vi "GetStatusParkerX.vi"(0 "Channel Properties":T1={"Channel Name"="", "Vel. Default"=5.0, "Acc. Default"=5.0, "Vel. Max"=5.0, "Vel. Min"=5.0, "Acc. Max"=5.0, "Acc. Min"=5.0, "Pulses/unit"=0.0, "Address"=0, "Pulse Offset"=0, "Pos Tolerance"=0.0, "Pulses/rev"=0.0, "Backlash/Eng units"=0.0, "Current Pos"=0.0, "Ch Status"=enum."Active", "Port Name"="", "Axis Transform mode"="", "Metadata Ch Name"="", "Type"=""} {"Current Pos" format="%.2f"; "Backlash/Eng units" format="%.2f"; "Pulses/rev" format="%.2f"; "Pos Tolerance" format="%.2f"; "Pulses/unit" format="%.2f"; "Acc. Min" format="%.2f"; "Acc. Max" format="%.2f"; "Vel. Min" format="%.2f"; "Vel. Max" format="%.2f"; "Acc. Default" format="%.2f"; "Vel. Default" format="%.2f"}, 2 "Limit switch valid?":bool, 3 "Stop on Trigger 3?":bool) -> (5 "Ready":bool, 6 "OK":bool, 7 "Position in Move":dbl format="%.2f", 8 "Error string":string)   [LabVIEW 2012]
uses:
  ~subVIs/DriveProperties.ctl
  X-_commands.ctl
panel:
  out "Output 2":i32
  out "Output 1":i32 format="%.0b"
  out "Remaining String":string
  out "CCW limit":bool
  out "Home":bool
  out "NOT FAULT":bool
  out "CCW limit":bool
  out "CW limit":bool
  out "Seq3":bool
  out "Seq2":bool
  out "Seq1":bool
  out "Trg3":bool
  out "Trg2":bool
  out "Trg1":bool
  out "Good Home":bool
  out "Stall":bool
  out "Trigger":bool
  out "Shutdown":bool
  out "Pausing":bool
  out "Looping":bool
  out "CW limit":bool
  out "Status":string
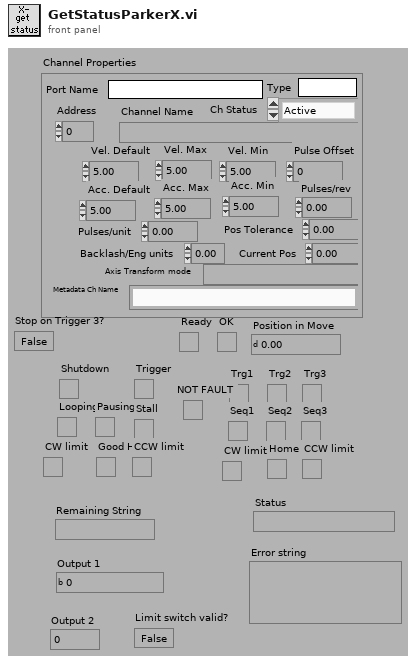
[diagram p1: front panel]
types:
  T1 = typedef "DriveProperties.ctl" = cluster{"Channel Name":string, "Vel. Default":dbl, "Acc. Default":dbl, "Vel. Max":dbl, "Vel. Min":dbl, "Acc. Max":dbl, "Acc. Min":dbl, "Pulses/unit":dbl, "Address":u8, "Pulse Offset":i32, "Pos Tolerance":dbl, "Pulses/rev":dbl, "Backlash/Eng units":dbl, "Current Pos":dbl, "Ch Status":enum16{"Active", "Offline", "Simulate"}, "Port Name":string, "Axis Transform mode":string, "Metadata Ch Name":string, "Type":string}
  T2 = typedef "X-_commands.ctl" = enum16{"A-    Acceleration (rps)", "B-    Buffer Status", "C-    Continue", "CG-  Correction Gain", "CR-  Cariage Return", "D-    Distance (pulses)", "DB-  Dead Band (encoder steps)", "DW- Deadband Window (encoder steps)", "E-    Enable Communications", "ER-  Encoder Resolution (steps/rev)", "F-    Disable Communications", "FS-  Encoder Functions Report", "FSA- Incremental/Absolute (0/1)", "FSB- Motor/Encoder Step Mode (0/1)", "FSC- Enable/Disable Position Maint. (1/0)", "FSD- Stop/Continue on Stall (1/0)", "FSE- Activate o/p1 on Stall (1/0)", "FSF- Stop Motion on Trig3 (1/0)", "FSG- Activate o/p2 in Deadband (1/0)", "FSH- Enable Stall Detect (1/0)", "G- Go", "GH- Go Home and Zero (+/-V)", "^H- Delete ", "H- Direction Reverse/CCW/CW (0,1,2)", "IS- Input Status", "K- Kill", "L- Loop (n)", "LD- Limit DISABLE (0-none,1-CW,2-CCW,3-Both)", "LF- Line Feed", "MC- Mode Continuous", "MN- Mode Normal", "MPA- Motor Postion Absolute", "MPI- Motor Position Incremental", "MR- Motor Resolution (Drive Steps/rev)", "N- End of Loop", "O- Output (00,01,10,11)", "OS- Report Homing Setup", "OSA- NO/NC Limits (1/0)", "OSB- Back Up to Home/Edge? (0/1)", "OSC- NO/NC Home Switch (1/0)", "OSD- Enable Encoder Z for Home (0/1)", "OSH- Reference Edge for Home CW/CCW (0/1)", "PR- Report ABSOLUTE Position", "PS- Pause until Continue", "PX- Report Absolute ENCODER Position", "PZ- Zero Absolute Counter", "\"- Quote (17 ASCII +Space)", "Q- Enter/Exit Velocity Profiling (1/0)", "R- Request Indexer Status", "RA- Report Limit Switch Status", "RB- Report Loop, Pause, Shutdown, Trigger Status", "RC- Report Closed Loop Status", "RM- Velocity Streaming Rate Multiplier (000-FFF)", "RV- Report Revision Level", "S- Controlled Stop", "SN- Debounce (1-1000ms)", "SS- Report Software Switch Status", "SSA- Disable RS232 Echo (1/0)", "SSG- Clear/Save Command Buffer on Limit (0/1)", "SSH- Clear/Save Command Buffer on Stop (0/1)", "ST- Shutdown (1/0)", "SV- Servoing Setting (0,1,2,3)", "T- Time Delay (0.01-99999.99)", "TR- Wait for Trigger High/Low/Ignore (1/0/X)", "TS- Report Trigger Status", "U- Pause after Move Until Continue", "V- Velocity (0.01-50.00 revs/sec)", "W1- Report Relative Position <Signed Binary>", "W3- Report Relative Position <Hexadecimal>", "Y- Abort Loop at N", "Z-    Reset to Defaults", "#-    Disable/Set Soft Addresses (0/1-255)"}
  T3 = cluster{"Boolean array[0]":bool, "Boolean array[1]":bool, "Boolean array[2]":bool, "Boolean array[3]":bool}
  T4 = cluster{"Boolean array[0]":bool, "Boolean array[1]":bool, "Boolean array[2]":bool, "Boolean array[3]":bool, "Boolean array[4]":bool, "Boolean array[5]":bool, "Boolean array[6]":bool, "Boolean array[7]":bool, "Boolean array[8]":bool, "Boolean array[9]":bool}
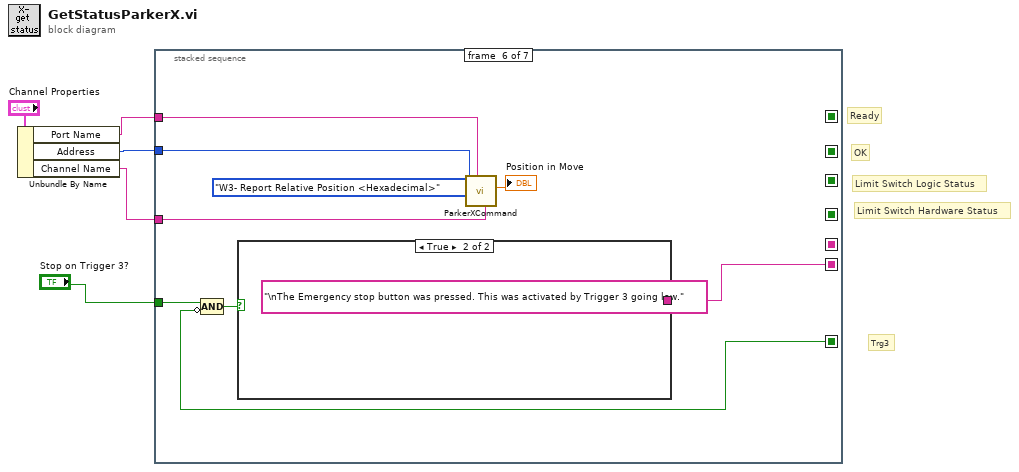
[diagram p0: block diagram]
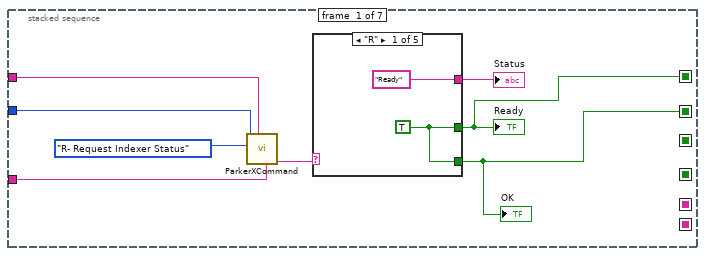
[diagram p2: hidden frame]
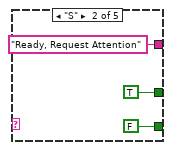
[diagram p3: hidden frame]
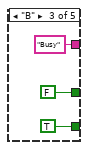
[diagram p4: hidden frame]
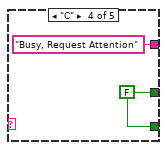
[diagram p5: hidden frame]
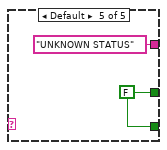
[diagram p6: hidden frame]
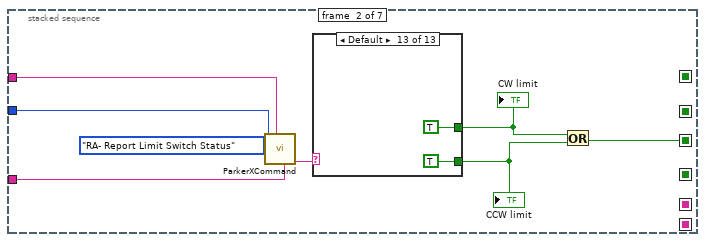
[diagram p7: hidden frame]
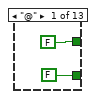
[diagram p8: hidden frame]
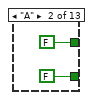
[diagram p9: hidden frame]
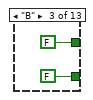
[diagram p10: hidden frame]
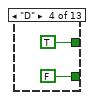
[diagram p11: hidden frame]
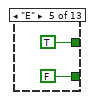
[diagram p12: hidden frame]
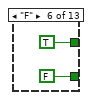
[diagram p13: hidden frame]
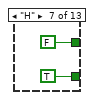
[diagram p14: hidden frame]
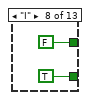
[diagram p15: hidden frame]
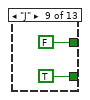
[diagram p16: hidden frame]
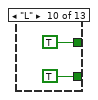
[diagram p17: hidden frame]
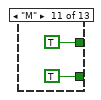
[diagram p18: hidden frame]
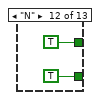
[diagram p19: hidden frame]
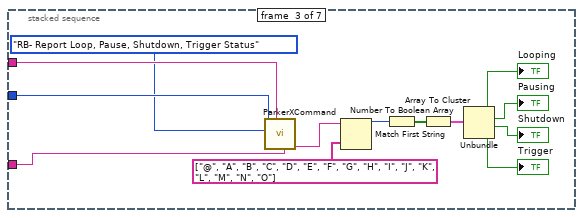
[diagram p20: hidden frame]
diagram:
  # "Trg3"
  # "Limit Switch Hardware Status"
  # "Limit Switch Logic Status"
  # "Ready"
  # "OK"
  n1 = Unbundle By Name("Channel Properties") -> ("Port Name"=w5:string, "Address"=w4:u8, "Channel Name"=w3:string)
  n2 = stacked-sequence {
    seq-local: [_ _ _ _ w94 _ _] -> [_ _ _ _ _ _ w138]
    seq-local: [_ w26 _ _ _ _ _] -> [_ _ _ _ _ _ w139]
    seq-local: [w8 _ _ _ _ _ _] -> [_ _ _ _ _ _ _]
    seq-local: [_ _ _ w73 _ _ _] -> [_ _ _ _ _ _ w146]
    seq-local: [w6 _ _ _ _ _ _] -> [_ _ _ _ _ _ w140]
    seq-local: [_ _ _ _ w93 _ _] -> [_ _ _ _ _ w126 _]
    seq-local: [_ _ _ _ _ w128 _] -> [_ _ _ _ _ _ w136]
    tunnel: w4 -> [w13 w33 w72 w82 w97 w133 _]
    tunnel: w5 -> [w7 w32 w71 w81 w96 w132 _]
    tunnel: w3 -> [w9 w29 w60 w77 w95 w129 w141]
    tunnel: "Stop on Trigger 3?" -> [_ _ _ _ w92 w127 _]
    frame #0 {
      n3 = call "ParkerXCommand.vi"("Channel Name"=w9, "Port Name"=w7, "COMMAND"=X-_commands."R- Request Indexer Status", "Address"=w13) -> ("String Reply"=w12:string)  [unwired: 3 in, 3 out]
      n4 = case shown="\"R\"" w12 {
        tunnel: ["Ready" "Ready, Request Attention" "Busy" "Busy, Request Attention" "UNKNOWN STATUS"] -> w11
        tunnel: [w14 TRUE FALSE w22 w24] -> w6
        tunnel: [w14 FALSE TRUE w22 w24] -> w8
        frame "R" {
          w14 = TRUE
        }
        frame "S" {
        }
        frame "B" {
        }
        frame "C" {
          w22 = FALSE
        }
        frame Default {
          w24 = FALSE
        }
      }
      "Status" <- w11
      "Ready" <- w6
      "OK" <- w8
    }
    frame #1 {
      n5 = call "ParkerXCommand.vi"("Channel Name"=w29, "Port Name"=w32, "COMMAND"=X-_commands."RA- Report Limit Switch Status", "Address"=w33) -> ("String Reply"=w31:string)  [unwired: 3 in, 3 out]
      n6 = case shown="Default" w31 {
        tunnel: [FALSE FALSE FALSE TRUE TRUE TRUE FALSE FALSE FALSE TRUE TRUE TRUE TRUE] -> w28
        tunnel: [FALSE FALSE FALSE FALSE FALSE FALSE TRUE TRUE TRUE TRUE TRUE TRUE TRUE] -> w27
        frame "@" {
        }
        frame "A" {
        }
        frame "B" {
        }
        frame "D" {
        }
        frame "E" {
        }
        frame "F" {
        }
        frame "H" {
        }
        frame "I" {
        }
        frame "J" {
        }
        frame "L" {
        }
        frame "M" {
        }
        frame "N" {
        }
        frame Default {
        }
      }
      "CW limit" <- w28
      "CCW limit" <- w27
      n7 = Or(x=w28, y=w27) -> (x .or. y?=w26:bool)
    }
    frame #2 {
      n8 = call "ParkerXCommand.vi"("Channel Name"=w60, "Port Name"=w71, "COMMAND"=X-_commands."RB- Report Loop, Pause, Shutdown, Trigger Status", "Address"=w72) -> ("String Reply"=w69:string)  [unwired: 3 in, 3 out]
      n9 = Match First String(2:string[] ["@", "A", "B", "C", "D", "E", "F", "G", "H", "I", "J", "K", "L", "M", "N", "O"], 3:w69) -> (0:w67:i32)  [unwired: 1 out]
      n10 = Number To Boolean Array(number=w67) -> (Boolean array=w66:bool[])
      n11 = Array To Cluster(array=w66) -> (cluster=w65:T3)
      n12 = Unbundle(w65) -> ("Boolean array[0]"=→"Looping":bool, "Boolean array[1]"=→"Pausing":bool, "Boolean array[2]"=→"Shutdown":bool, "Boolean array[3]"=→"Trigger":bool)
    }
    frame #3 {
      n13 = call "ParkerXCommand.vi"("Channel Name"=w77, "Port Name"=w81, "COMMAND"=X-_commands."RC- Report Closed Loop Status", "Address"=w82) -> ("String Reply"=w79:string)  [unwired: 3 in, 3 out]
      n14 = case shown="\"B\"" w79 {
        tunnel: [FALSE TRUE FALSE TRUE w91] -> w74
        tunnel: [TRUE TRUE FALSE FALSE w91] -> w78
        frame "@" {
        }
        frame "A" {
        }
        frame "B" {
        }
        frame "C" {
        }
        frame Default {
          w91 = FALSE
          (unwired) "UNKNOWN STATUS"
        }
      }
      "Stall" <- w74
      "Good Home" <- w78
      n15 = Select(t=" Motor Stalled", s=w74, f="") -> (s? t:f=w73:string)
    }
    frame #4 {
      n16 = while {
        tunnel: w97 -> [w124]
        tunnel: w96 -> [w123]
        tunnel: w95 -> [w121]
        tunnel: [w104] -> w94
        tunnel: [w103] -> w93
        tunnel: w92 -> [w98]
        i -> [w102]
        stop <- w99 continue-if-true
        n17 = call "ParkerXCommand.vi"("Channel Name"=w121, "Port Name"=w123, "COMMAND"=X-_commands."IS- Input Status", "Address"=w124) -> ("String Reply"=w120:string)  [unwired: 3 in, 3 out]
        n18 = Scan From String(format string="%10b%1d" ("Format String"), input string=w120) -> (remaining string=→"Remaining String":string, output 1=w116:i32, output 2=→"Output 2":i32)  [unwired: 2 in, 4 out]
        "Output 1" <- w116
        n19 = Less?(x=w102, y=3) -> (x < y?=w100:bool)
        n20 = Number To Boolean Array(number=w116) -> (Boolean array=w115:bool[])
        n21 = Array To Cluster(array=w115) -> (cluster=w114:T4)
        n22 = Unbundle(w114) -> ("Boolean array[0]"=→"Seq3":bool, "Boolean array[1]"=→"Seq2":bool, "Boolean array[2]"=→"Seq1":bool, "Boolean array[3]"=w106:bool, "Boolean array[4]"=w105:bool, "Boolean array[5]"=→"NOT FAULT":bool, "Boolean array[6]"=→"Home":bool, "Boolean array[7]"=w103:bool, "Boolean array[8]"=→"Trg2":bool, "Boolean array[9]"=→"Trg1":bool)
        "Trg3" <- w103
        "CCW limit" <- w105
        "CW limit" <- w106
        n23 = Or(x=w106, y=w105) -> (x .or. y?=w104:bool)
        n24 = Compound Arithmetic op=AND(w98, invert w103, w100) -> (w99:bool)
      }
    }
    frame #5 {
      n25 = Compound Arithmetic op=AND(w127, invert w126) -> (w125:bool)
      n26 = case shown="True" w125 {
        tunnel: ["" "\nThe Emergency stop button was pressed. This was activated by Trigger 3 going low."] -> w128
        frame False {
        }
        frame True {
        }
      }
      n27 = call "ParkerXCommand.vi"("Channel Name"=w129, "Port Name"=w132, "COMMAND"=X-_commands."W3- Report Relative Position <Hexadecimal>", "Address"=w133) -> ("Numeric Reply"=→"Position in Move":dbl)  [unwired: 3 in, 3 out]
    }
    frame #6 {
      n28 = Compound Arithmetic op=AND("Limit switch valid?", w138, w139, w140) -> (w145:bool)
      n29 = Select(t=" Hit limit switch. ", s=w145, f="") -> (s? t:f=w147:string)
      n30 = Concatenate Strings(w136, w146, w147) -> (w142:string)
      n31 = Empty String/Path?(string/path=w142) -> (empty?=w144:bool)
      n32 = case shown="False" w144 {
        tunnel: [w150 w153] -> w143
        tunnel: w142 -> [w151 w153]
        tunnel: w141 -> [w152 _]
        frame False {
          n33 = Concatenate Strings(w152, w151) -> (w150:string)
        }
        frame True {
        }
      }
      "Error string" <- w143
    }
  }
